vi "Main.vi"(11 "Module Admin":refnum<class "Delacor_lib_QMH_Module Admin.lvclass">) -> ()   [LabVIEW 2020, in "Cycling by State module.lvlib"]
doc: "This template is based off of the Queued Message Handler design pattern and the Queued Message Handler project template that ships with LabVIEW.\n\nThe main difference is that the queue is private to this module and communication between modules is performed via Broadcast and Request events.\n\nRequest events are wrapped in public API methods and are handled in the Event Handling Loop (EHL) of this VI. Any module can register for Broadcast events sent by this module. The EHL generates messages based on user interface actions.\n\nThe Message Handling Loop (MHL) processes messages generated by the EHL, or by other messages. The messages are string values, so new messages can be added easily to the Message Cases case structure in the MHL. Each message cluster can also provide an optional value for Message Data, which is a variant that can be converted to whatever message-specific data is required.\n_____\nBased on DQMH Project Template 7.0.1.1316."
uses:
  Cycling by State module.lvlib
  <vilib>/Delacor/Delacor QMH/Libraries/Module Admin_class/Delacor_lib_QMH_Module Admin.lvclass
  Module Data--cluster.ctl
  Cycling HL Data--cluster.ctl
  Cycling state.ctl
  <vilib>/Delacor/Delacor QMH/Libraries/Message Queue_class/Delacor_lib_QMH_Message Queue.lvclass/Delacor_lib_QMH_Message Queue.ctl
  Stop Argument--cluster.ctl
  <vilib>/Delacor/Delacor QMH/Libraries/Module Admin_class/Delacor_lib_QMH_Module Admin.lvclass/Delacor_lib_QMH_Module Admin.ctl
  Start cycling Argument--cluster.ctl
  Stop cycling Argument--cluster.ctl
  <vilib>/Utility/miscctls.llb/LVPointTypeDef.ctl
  <vilib>/Delacor/Delacor QMH/Libraries/Message Queue_class/Delacor_lib_QMH_Enqueue Message (Single).vi
  <vilib>/Delacor/Delacor QMH/Libraries/Module Admin_class/Delacor_lib_QMH_Get External Launch.vi
  <vilib>/Delacor/Delacor QMH/Libraries/Message Queue_class/Delacor_lib_QMH_Message Queue.lvclass
  Sensor checking module/Sensor checking module.lvlib
panel:
  out "error out":errorcluster
  out "Status":string
  in  "Simulate MHL Error":bool
  in  "Simulate EHL Error":bool
  # "Other processes communicate with this Module via its Public API (wrappers for its Request Events).\n\nThis Module communicates with other processes via its Broadcast Events.\nAny process that wants to receive these messages can register for this module's Broadcast events."
  # "This template is for the DQMH framework. See the block diagram for more information on how to use this template."
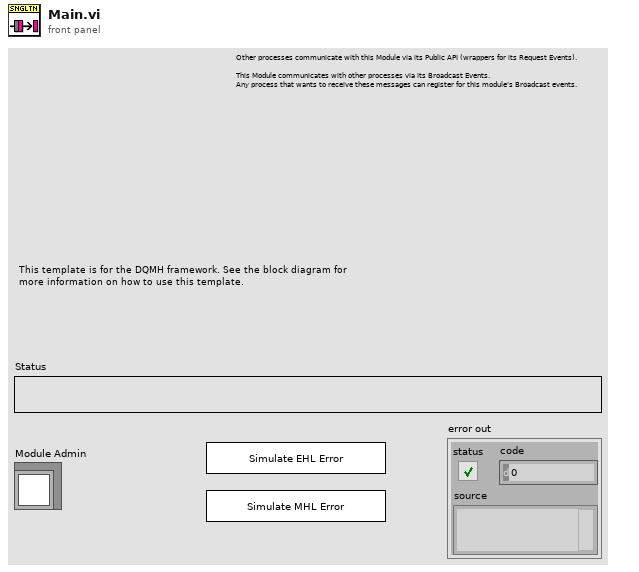
[diagram p1: front panel]
types:
  T1 = typedef "Cycling by State module.lvlib/Request Events--cluster.ctl" = cluster{"Stop Module":refnum<user-event>, "Show Panel":refnum<user-event>, "Hide Panel":refnum<user-event>, "Get Module Execution Status":refnum<user-event>, "Show Diagram":refnum<user-event>, "Start cycling":refnum<user-event>, "Stop cycling":refnum<user-event>, "Private":cluster{"Wake up cycling HL":refnum<user-event>}, "Put Cycling HL to sleep":refnum<user-event>}
  T2 = typedef "Sensor checking module.lvlib/Broadcast Events--cluster.ctl" = cluster{"Module Did Init":refnum<user-event>, "Status Updated":refnum<user-event>, "Error Reported":refnum<user-event>, "Module Did Stop":refnum<user-event>, "Update Module Execution Status":refnum<user-event>, "Triggered Broadcast":refnum<user-event>}
  T3 = typedef "Cycling by State module.lvlib/Cycling HL Data--cluster.ctl" = cluster{"Enum":T4, "RPM":dbl, "Triggered interval":dbl}
  T4 = typedef "Cycling state.ctl" = enum16{"Accelerating to 110rpm", "Detecting 100rpm", "Pressing until 0rpm"}
  T5 = typedef "Cycling by State module.lvlib/Module Data--cluster.ctl" = cluster{"Status":string}
  T6 = enum32{"invalid lock state", "Not Locked", "Locked (No Password)", "Password-protected"}
  T7 = typedef "Cycling by State module.lvlib/Stop Argument--cluster.ctl" = cluster{"Origin":string, "Exit via Stop Module Req?":bool, "Wait for Module to stop?":bool}
  T8 = typedef "Cycling by State module.lvlib/Start cycling Argument--cluster.ctl" = cluster{"Triggered interval":dbl, "Cycling interval":dbl}
  T9 = typedef "Cycling by State module.lvlib/Stop cycling Argument--cluster.ctl" = cluster{"Boolean":bool}
  T10 = typedef "LVPointTypeDef.ctl" = cluster{"Horizontal":i16, "Vertical":i16}
  T11 = enum32{"Invalid", "Standard", "Closed", "Hidden", "Minimized", "Maximized"}
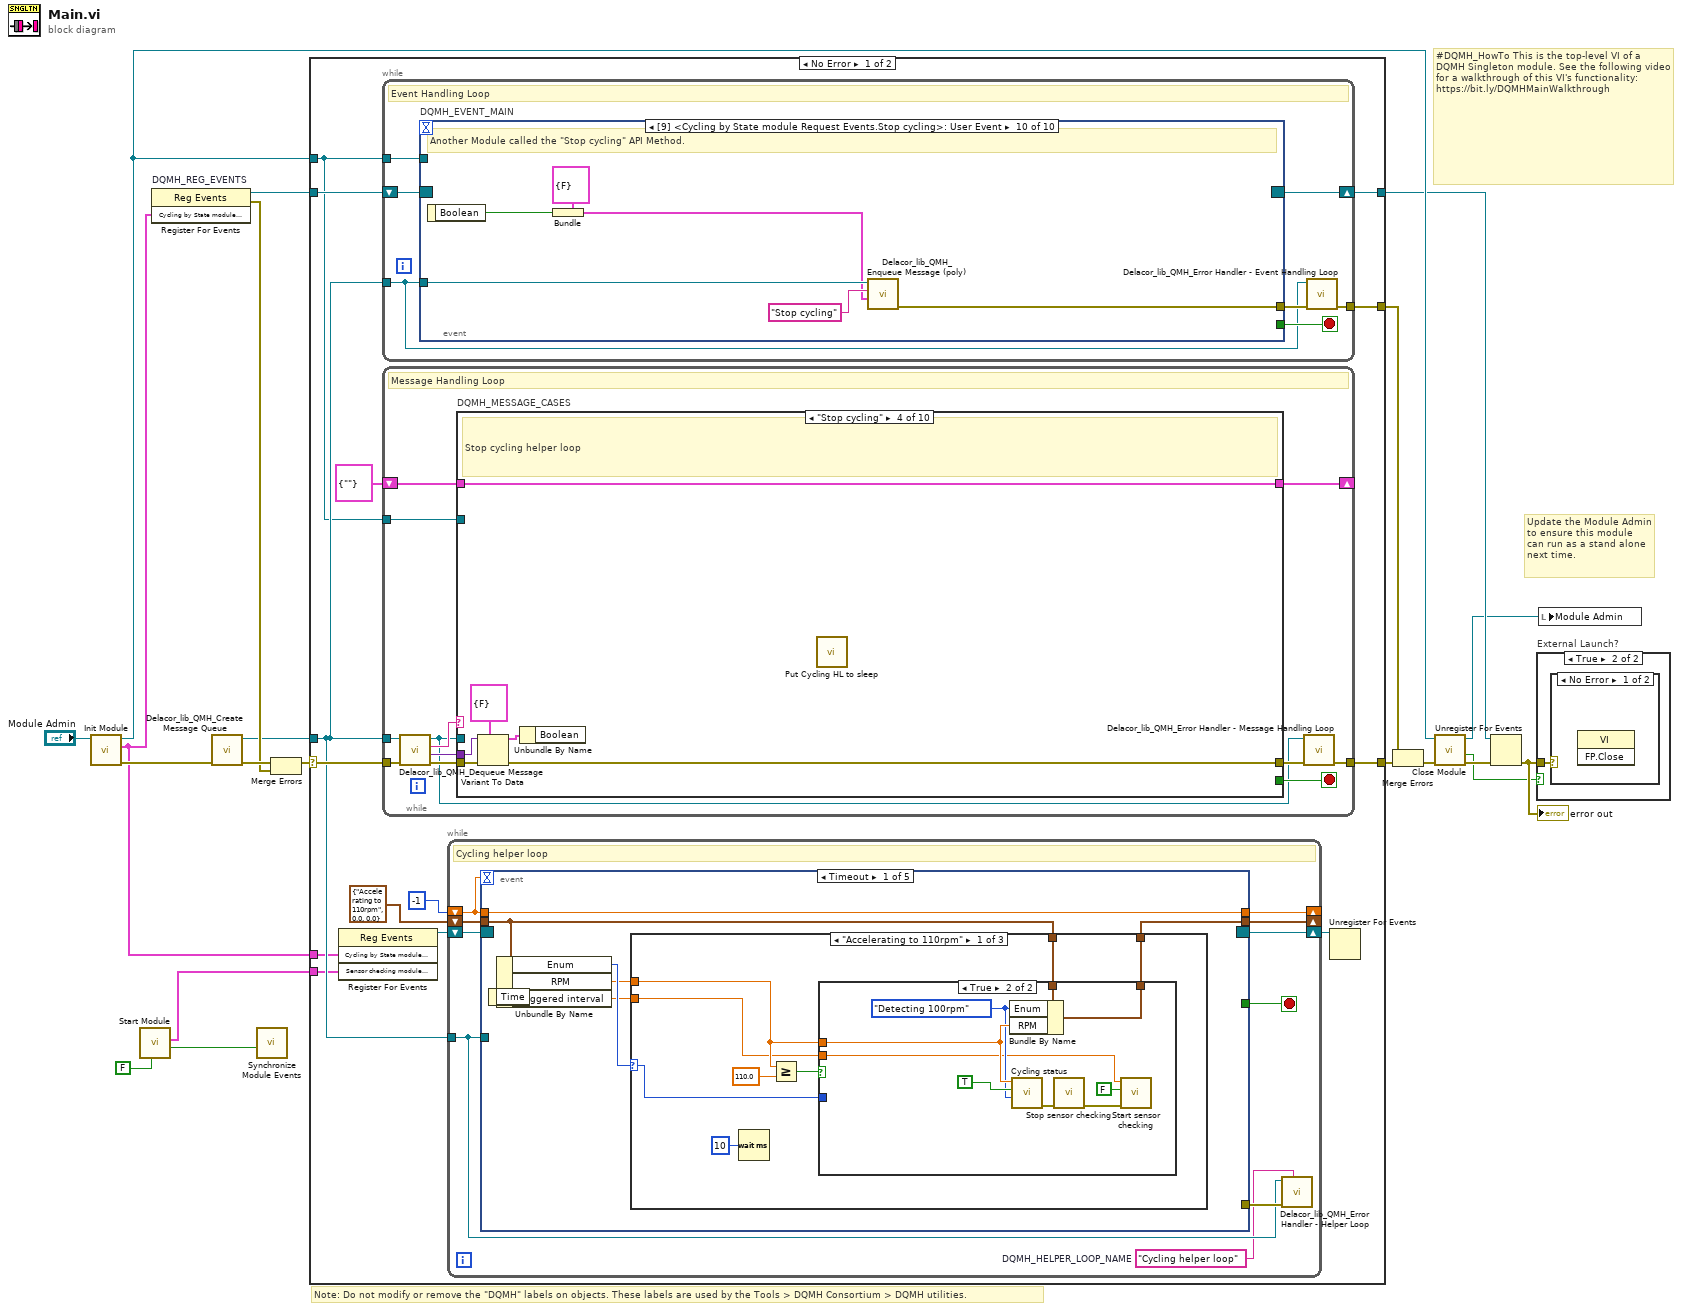
[diagram p0: block diagram]
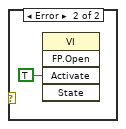
[diagram p3: hidden frame]
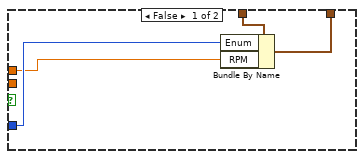
[diagram p4: hidden frame]
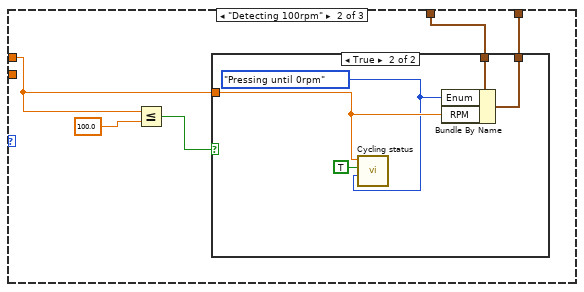
[diagram p5: hidden frame]
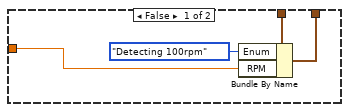
[diagram p6: hidden frame]
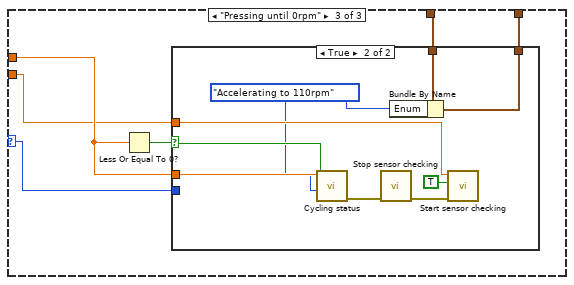
[diagram p7: hidden frame]
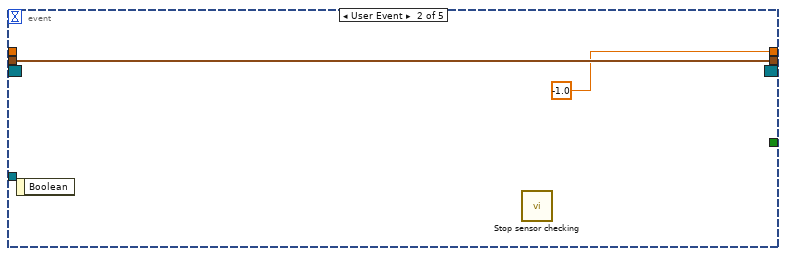
[diagram p9: hidden frame]
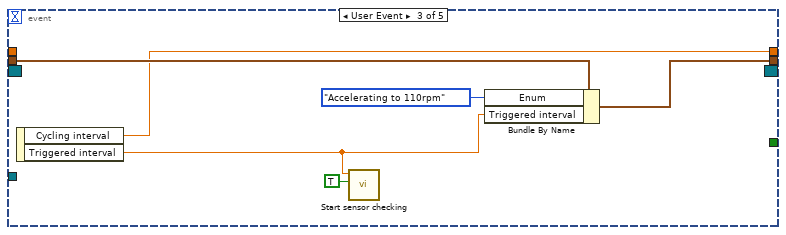
[diagram p10: hidden frame]
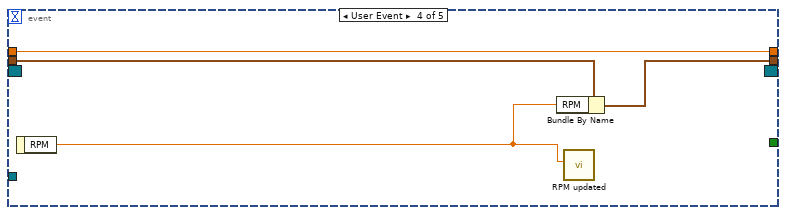
[diagram p11: hidden frame]
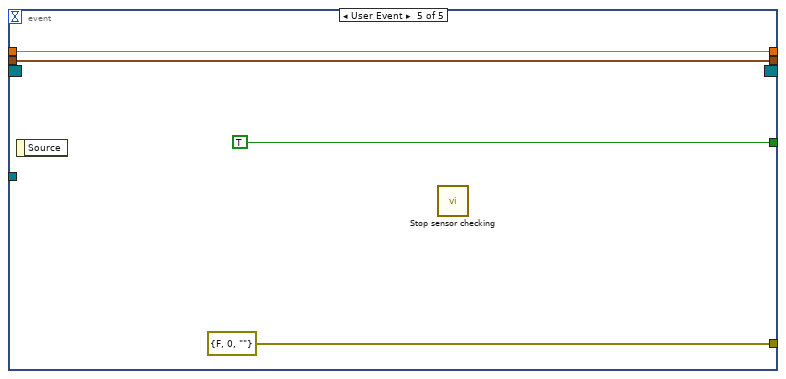
[diagram p12: hidden frame]
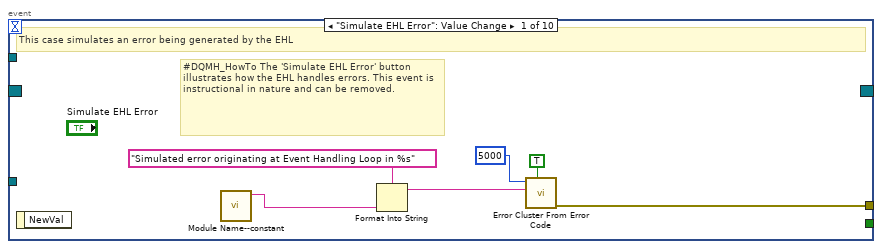
[diagram p13: hidden frame]
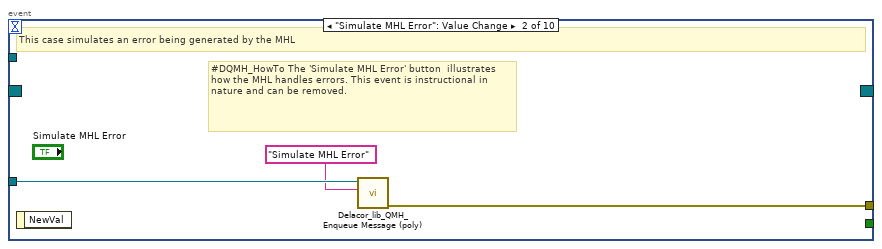
[diagram p14: hidden frame]
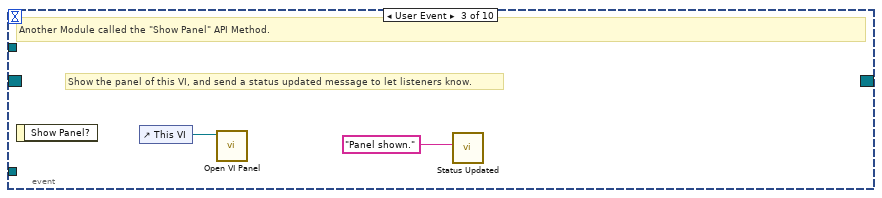
[diagram p15: hidden frame]
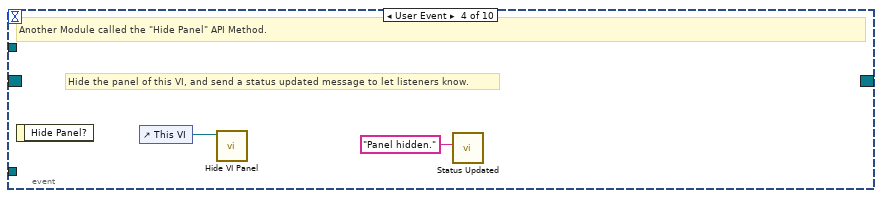
[diagram p16: hidden frame]
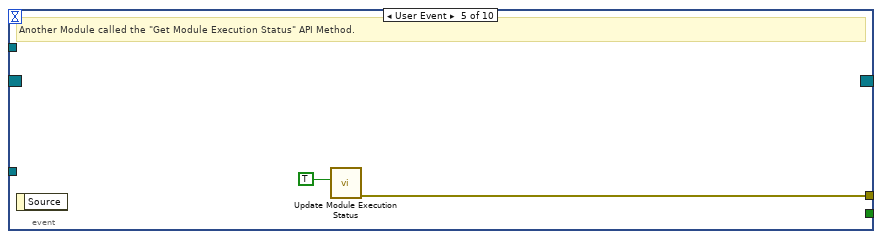
[diagram p17: hidden frame]
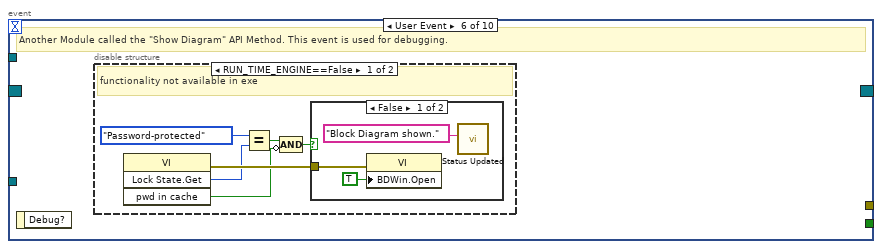
[diagram p18: hidden frame]
diagram:
  # "#DQMH_HowTo This is the top-level VI of a DQMH Singleton module. See the following video for a walkthrough of this VI's functionality: https://bit.ly/DQMHMainWalkthrough"
  # "Note: Do not modify or remove the \"DQMH\" labels on objects. These labels are used by the Tools > DQMH Consortium > DQMH utilities."
  # "Update the Module Admin to ensure this module can run as a stand alone next time."
  n1 = call "Init Module.vi"("Singleton Module Admin in"="Module Admin") -> ("error out"=w19:errorcluster, "Cycling by State module Request Events"=w3:T1, "Singleton Module Admin out"=w11:refnum<class "Delacor_lib_QMH_Module Admin.lvclass">)  [unwired: 8 in]
  n2 = call "Start Module.vi"("Show Main VI Diagram on Init (F)"=FALSE) -> ("Wait for Event Sync?"=w1:bool, "Sensor checking module Broadcast Events"=w2:T2)  [unwired: 7 in, 2 out]
  n3 = register-events "DQMH_REG_EVENTS"(w3) -> (reference out=w9:refnum<event-registration>, error out=w12:errorcluster)  [unwired: 2 in]
  n4 = call <vilib>:"Delacor_lib_QMH_Create Message Queue.vi"("error in"=w19) -> ("error out"=w14:errorcluster, "Message Queue"=w8:refnum<class "Delacor_lib_QMH_Message Queue.lvclass">)  [unwired: 9 in]
  n5 = call "Synchronize Module Events.vi"("Wait for Event Sync?"=w1) -> ()  [unwired: 10 in, 1 out]
  n6 = Merge Errors(w14, w12) -> (w13:errorcluster)
  n7 = case shown="No Error" w13 {
    selector: w13 -> [w32 w297]
    tunnel: [w34 w296] -> w20
    tunnel: [w31 w295] -> w10
    tunnel: w9 -> [w29 w295]
    tunnel: w8 -> [w28 w290]
    tunnel: [w33 _] -> w17
    tunnel: w11 -> [w27 w291]
    tunnel: w3 -> [w26 _]
    tunnel: w2 -> [w22 _]
    frame No Error {
      n8 = register-events ("DQMH_HELPER_REGFOREVENTS")(w26, w22) -> (reference out=w24:refnum<event-registration>)  [unwired: 2 in, 1 out]
      n9 = while {
        tunnel: w28 -> [w118]
        shift-right: [w121] -> w31
        shift-left: w29 -> [w122]
        tunnel: [w123] -> w33
        tunnel: w27 -> [w119]
        stop <- w120 stop-if-true
        # "Event Handling Loop"
        n10 = event "DQMH_EVENT_MAIN" shown="[9] <Cycling by State module Request Events.Stop cycling>: User Event" {
          selector: w122 -> [_ _ _ _ _ _ _ _ _ _]
          dyn-events: [_ _ _ _ _ _ _ _ _ _] -> w121
          timeout: _ -> [_ _ _ _ _ _ _ _ _ _]
          tunnel: [_ _ _ _ _ _ TRUE ("Discard?") _ _ _] -> w120
          tunnel: w118 -> [_ w132 _ _ _ _ w156 w163 w179 w185]
          tunnel: [w130 w133 _ _ w139 _ w159 w165 w174 w180] -> w124
          tunnel: w119 -> [_ _ _ _ _ _ _ w162 _ _]
          event "Simulate EHL Error": Value Change {
            # "#DQMH_HowTo The 'Simulate EHL Error' button  illustrates how the EHL handles errors. This event is instructional in nature and can be removed."
            # "This case simulates an error being generated by the EHL"
            n11 = event-data() -> ()  [unwired: 1 in, 1 out]
            n12 = call "Module Name--constant.vi"() -> ("Module Name"=w127:string)  [unwired: 11 in]
            n13 = Format Into String(format string="Simulated error originating at Event Handling Loop in %s", w127) -> (resulting string=w128:string)  [unwired: 2 in, 1 out]
            n14 = call <vilib>:"Error Cluster From Error Code.vi"("show call chain? (False)"=TRUE, "error message (\"\")"=w128, "error code (0)"=5000) -> ("error out"=w130:errorcluster)  [unwired: 6 in]
          }
          event "Simulate MHL Error": Value Change {
            # "#DQMH_HowTo The 'Simulate MHL Error' button  illustrates how the MHL handles errors. This event is instructional in nature and can be removed."
            # "This case simulates an error being generated by the MHL"
            n15 = event-data() -> ()  [unwired: 1 in, 1 out]
            n16 = call-poly <vilib>:"Delacor_lib_QMH_Enqueue Message (poly).vi"("Message"="Simulate MHL Error", "Message Queue in"=w132) -> ("error out"=w133:errorcluster)  [unwired: 8 in, 1 out]
          }
          event User Event {
            # "Show the panel of this VI, and send a status updated message to let listeners know."
            # "Another Module called the \"Show Panel\" API Method."
            n17 = event-data() -> ()  [unwired: 1 in, 1 out]
            n18 = control-ref of="This VI"() -> (w135:refnum<vi>)
            n19 = call "Open VI Panel.vi"("VI"=w135) -> ()  [unwired: 10 in, 1 out]
            n20 = call "Status Updated.vi"("Status"="Panel shown." ("format string")) -> ()  [unwired: 10 in, 1 out]
          }
          event User Event {
            # "Hide the panel of this VI, and send a status updated message to let listeners know."
            # "Another Module called the \"Hide Panel\" API Method."
            n21 = event-data() -> ()  [unwired: 1 in, 1 out]
            n22 = control-ref of="This VI"() -> (w137:refnum<vi>)
            n23 = call "Hide VI Panel.vi"("VI"=w137) -> ()  [unwired: 10 in, 1 out]
            n24 = call "Status Updated.vi"("Status"="Panel hidden." ("format string")) -> ()  [unwired: 10 in, 1 out]
          }
          event User Event {
            # "Another Module called the \"Get Module Execution Status\" API Method."
            n25 = event-data() -> ()  [unwired: 1 in, 1 out]
            n26 = call "Update Module Execution Status.vi"("Running?"=TRUE) -> ("error out"=w139:errorcluster)  [unwired: 10 in]
          }
          event User Event {
            # "Another Module called the \"Show Diagram\" API Method. This event is used for debugging."
            n27 = event-data() -> ()  [unwired: 1 in, 1 out]
            n28 = disable-structure shown="RUN_TIME_ENGINE==False" {
              frame condition #0 (active) {
                # "functionality not available in exe"
                n29 = invoke on="Invoke Node" class="VI" method="Lock State.Get"() -> (error out=w145:errorcluster, "Get Lock State"=w144:T6, "pwd in cache"=w141:bool)  [unwired: 4 in, 1 out]
                n30 = Equal?(x=T6."Password-protected", y=w144) -> (x = y?=w142:bool)
                n31 = Compound Arithmetic op=AND(w142, invert w141) -> (w140:bool)
                n32 = case shown="False" w140 {
                  tunnel: w145 -> [w148 _]
                  frame False {
                    n33 = property on="Property Node" class="VI"(error in=w148, "BDWin.Open"=TRUE ("Block Diagram Window:Open")) -> ()  [unwired: 1 in, 2 out]
                    n34 = call "Status Updated.vi"("Status"="Block Diagram shown." ("format string")) -> ()  [unwired: 10 in, 1 out]
                  }
                  frame True {
                    # "Password-protected VI, and the password is not in the cache. Do not show the diagram."
                  }
                }
              }
              frame condition #1 {
              }
            }
          }
          event User Event {
            # "The Stop Module Event can get fired from the Exit message in the MHL. The queue gets destroyed in that case. If the queue no longer exists, the Enqueue Exit as a priority message will return error 1. It is safe to ignore, because the module is already exiting."
            # "Another Module called the \"Stop Module\" API Method  or the Message Handling Loop below."
            n35 = event-data() -> ("Origin"=w155:string, "Exit via Stop Module Req?"=w151:bool, "Wait for Module to stop?"=w150:bool)  [unwired: 1 in]
            n36 = local write "Status"(w155) -> ()
            n37 = Bundle By Name(cluster=T7 {"Origin"="", "Exit via Stop Module Req?"=FALSE, "Wait for Module to stop?"=FALSE} ("Stop Argument"), "Exit via Stop Module Req?"=w151, "Wait for Module to stop?"=w150) -> (w149:T7)
            n38 = call-poly <vilib>:"Delacor_lib_QMH_Enqueue Message (poly).vi"("Priority Message? (F)"=TRUE, "Message Data"=w149, "Message"="Exit", "Message Queue in"=w156) -> ("error out"=w160:errorcluster)  [unwired: 6 in, 1 out]
            n39 = call <vilib>:"Clear Errors.vi"("error in (no error)"=w160, "specific error code to clear (0: all)"=1) -> ("error out"=w159:errorcluster)  [unwired: 4 in, 1 out]
          }
          event Panel Close? {
            w164 = TRUE  # Discard the event, the MHL is responsible for closing and stopping this VI.
            # "Hide the panel or send the 'Exit' message if the user clicks the 'X' on the module main VI panel."
            n40 = event-data() -> ()  [unwired: 1 in, 1 out]
            n41 = property on="Property Node" class="Module Admin"(reference=w162) -> ("Accessors:External Launch"=w161:bool)  [unwired: 1 in, 2 out]
            n42 = case shown="True" w161 {
              tunnel: w163 -> [_ w171]
              tunnel: [_ w172] -> w165
              frame True {
                # "If externally launched, clicking the 'X' hides the panel, but doesn't close it."
                n43 = control-ref of="This VI"() -> (w168:refnum<vi>)
                n44 = call "Hide VI Panel.vi"("VI"=w168) -> ("error out"=w166:errorcluster)  [unwired: 10 in]
                n45 = call "Status Updated.vi"("error in"=w166, "Status"="Panel hidden." ("format string")) -> ()  [unwired: 9 in, 1 out]
              }
              frame False {
                # "If run as a stand-alone VI, clicking the panel 'X' stops the VI."
                n46 = call-poly <vilib>:"Delacor_lib_QMH_Enqueue Message (poly).vi"("Priority Message? (F)"=TRUE, "Message"="Exit", "Message Queue in"=w171) -> ("error out"=w172:errorcluster)  [unwired: 7 in, 1 out]
              }
            }
            n47 = event-data ("Event Filter Node")("Discard?"=w164) -> ()  [unwired: 1 in, 1 out]
          }
          event User Event {
            # "Another Module called the \"Start cycling\" API Method."
            n48 = event-data() -> ("Triggered interval"=w175:dbl, "Cycling interval"=w173:dbl)  [unwired: 1 in]
            n49 = Bundle(cluster=T8 {"Triggered interval"=500.0, "Cycling interval"=500.0} ("Start cycling Argument"), "Triggered interval"=w175, "Cycling interval"=w173) -> (w176:T8)
            n50 = call-poly <vilib>:"Delacor_lib_QMH_Enqueue Message (poly).vi"("Message Data"=w176, "Message"="Start cycling", "Message Queue in"=w179) -> ("error out"=w174:errorcluster)  [unwired: 7 in, 1 out]
          }
          event User Event {
            # "Another Module called the \"Stop cycling\" API Method."
            n51 = event-data() -> ("Boolean"=w181:bool)  [unwired: 1 in]
            n52 = Bundle(cluster=T9 {"Boolean"=FALSE} ("Stop cycling Argument"), "Boolean"=w181) -> (w182:T9)
            n53 = call-poly <vilib>:"Delacor_lib_QMH_Enqueue Message (poly).vi"("Message Data"=w182, "Message"="Stop cycling", "Message Queue in"=w185) -> ("error out"=w180:errorcluster)  [unwired: 7 in, 1 out]
          }
        }
        n54 = call-dynamic "Delacor_lib_QMH_Error Handler - Event Handling Loop.vi"("error in"=w124, "Message Queue in"=w118) -> ("dup error in"=w123:errorcluster)  [unwired: 8 in, 1 out]
      }
      n55 = while {
        tunnel: w28 -> [w186]
        shift-right: [w194] -> _
        shift-left: T5 {"Status"=""} ("Data Cluster") -> [w195]
        tunnel: w32 -> [w197]
        tunnel: [w189] -> w34
        tunnel: w27 -> [w190]
        stop <- w193 stop-if-true
        # "Message Handling Loop"
        n56 = call-dynamic "Delacor_lib_QMH_Dequeue Message.vi"("error in"=w197, "Message Queue in"=w186) -> ("error out"=w196:errorcluster, "Message Data"=w191:variant, "Message"=w192:string, "Message Queue out"=w187:refnum<class "Delacor_lib_QMH_Message Queue.lvclass">)  [unwired: 6 in]
        n57 = case "DQMH_MESSAGE_CASES" shown="\"Stop cycling\"" w192 {
          selector: w192 -> [_ _ _ _ _ _ _ _ _ w285]
          tunnel: w187 -> [_ _ _ _ _ _ _ w251 w273 _]
          tunnel: w196 -> [w215 w219 w227 w233 w236 w238 w247 w258 w279 w288]
          tunnel: [w213 w219 w225 w231 w235 w238 w246 w254 w274 w289] -> w188
          tunnel: w195 -> [w204 w218 w226 w232 w234 w237 w244 w253 w272 w286]
          tunnel: [w203 w218 w226 w232 w234 w237 w244 w253 w272 w286] -> w194
          tunnel: [_ _ _ _ _ _ _ _ w271 _] -> w193
          tunnel: w191 -> [_ _ w224 w230 _ _ _ w252 w270 _]
          tunnel: w190 -> [w205 _ _ _ _ _ _ w250 w265 _]
          frame "Initialize" {
            w199 = "Initial Message" ("Initial Message")
            # "#CodeNeeded - Initialize the appearance of the front panel."
            # "#CodeNeeded - Initialize your state data here."
            # "Initialize - Any operation that needs to be done before the module can receive messages. Synchronize Caller Events.vi will inform Start Module.vi that the module has launched and is ready to receive messages. Module Did Init.vi will broadcast that the module initialized."
            n58 = call "Synchronize Caller Events.vi"("error in"=w215, "Singleton Module Admin in"=w205) -> ("error out"=w214:errorcluster, "Singleton Module Admin out"=w200:refnum<class "Delacor_lib_QMH_Module Admin.lvclass">)  [unwired: 8 in]
            n59 = property on="Property Node" class="Module Admin"(reference=w200) -> ("Accessors:External Launch"=w209:bool)  [unwired: 1 in, 2 out]
            n60 = Select(t=T11."Hidden" ("State"), s=w209, f=T11."Standard" ("State")) -> (s? t:f=w206:T11)
            n61 = call "Module Name--constant.vi"() -> ("Module Name"=w212:string)  [unwired: 11 in]
            n62 = property on="Property Node" class="VI"("Front Panel.Title"=w212) -> (reference out=w211:refnum<vi>, error out=w217:errorcluster)  [unwired: 2 in]
            n63 = call "Module Name--constant.vi"() -> ("Module Name"=w201:string)  [unwired: 11 in]
            n64 = invoke on="Invoke Node" class="VI" method="FP.Open"(reference=w211, error in=w217, "State"=w206) -> (reference out=w210:refnum<vi>, error out=w216:errorcluster)  [unwired: 2 in, 3 out]
            n65 = Bundle By Name(cluster=w204, "Status"=w199) -> (w203:T5)
            n66 = call "Module Did Init.vi"("error in"=w214, "Initialized?"=TRUE, "Origin"=w201) -> ("error out"=w213:errorcluster)  [unwired: 8 in]
            n67 = invoke on="Invoke Node" class="VI" method="FP.Center"(reference=w210, error in=w216) -> ()  [unwired: 1 in, 3 out]
            n68 = property on="Pane" class="Pane"("Origin"=T10 {"Horizontal"=0, "Vertical"=0}) -> ()  [unwired: 2 in, 2 out]
            "Status" <- w199
          }
          frame "---Module Specific---" {
            # "Separator -- The following cases handle messages specific to this Module."
          }
          frame "Start cycling" {
            # "To start cycling by waking up cycling helper loop"
            n69 = Variant To Data(error in=w227, type=T8 {"Triggered interval"=500.0, "Cycling interval"=500.0} ("Start cycling Argument"), Variant=w224) -> (data=w222:T8, error out=w225:errorcluster)
            n70 = Unbundle By Name(w222) -> ("Triggered interval"=w221:dbl, "Cycling interval"=w220:dbl)
            n71 = call "Wake up cycling HL.vi"("Triggered interval"=w221, "Cycling interval"=w220) -> ()  [unwired: 8 in, 1 out]
          }
          frame "Stop cycling" {
            # "Stop cycling helper loop"
            n72 = Variant To Data(error in=w233, type=T9 {"Boolean"=FALSE} ("Stop cycling Argument"), Variant=w230) -> (data=w228:T9, error out=w231:errorcluster)
            n73 = Unbundle By Name(w228) -> ()  [unwired: 1 out]
            n74 = call "Put Cycling HL to sleep.vi"() -> ()  [unwired: 11 in, 1 out]
          }
          frame "---Copy This Frame---" {
            # "Duplicate this frame when creating new messages.  Change this comment in the duplicated frame to describe this message."
            n75 = Merge Errors(w236) -> (w235:errorcluster)
          }
          frame "---Exit and Error Handling---" {
            # "Separator - The following cases handle errors and exit messages."
          }
          frame "Simulate MHL Error" {
            # "#DQMH_HowTo The 'Simulate MHL Error' button  illustrates how the MHL handles errors. This event is instructional in nature and can be removed."
            # "Simulate an error occurring at the MHL"
            n76 = call "Module Name--constant.vi"() -> ("Module Name"=w240:string)  [unwired: 11 in]
            n77 = Format Into String(format string="Simulated error originating at Message Handling Loop in %s", w240) -> (resulting string=w241:string)  [unwired: 2 in, 1 out]
            n78 = call <vilib>:"Error Cluster From Error Code.vi"("show call chain? (False)"=TRUE, "error message (\"\")"=w241, "error code (0)"=5001) -> ("error out"=w245:errorcluster)  [unwired: 6 in]
            n79 = Merge Errors(w247, w245) -> (w246:errorcluster)
          }
          frame "Error" {
            # "#CodeRecommended - If the module is running in standalone mode (External Launch = FALSE), this code will pop up an error dialog and call the 'Exit' message if an error occurs. Add more fine-grained error management here."
            # "Error - Check the error message data and respond accordingly. This message is sent by the \"Error Handler\" VIs at the end of each loop in this application."
            n80 = property on="Property Node" class="Module Admin"(reference=w250) -> ("Accessors:External Launch"=w249:bool)  [unwired: 1 in, 2 out]
            n81 = Variant To Data(error in=w258, type=errorcluster {"status"=FALSE, "code"=0, "source"=""} ("error constant"), Variant=w252) -> (data=w248:errorcluster, error out=w256:errorcluster)
            n82 = local write "error out"(w248) -> ()
            n83 = call "Error Reported.vi"("Error"=w248) -> ()  [unwired: 10 in, 1 out]
            n84 = case shown="False" w249 {
              tunnel: [w263 _] -> w255
              tunnel: w251 -> [w261 _]
              tunnel: w248 -> [w262 _]
              frame False {
                n85 = disable-structure shown="Default" {
                  disable-tunnel: w262 -> [w264 _]
                  frame condition #0 (active) {
                    # "If the module is running standalone, then pop up an error dialog and call the \"Exit\" message."
                    n86 = call <vilib>:"Simple Error Handler.vi"("error in (no error)"=w264) -> ()  [unwired: 4 in, 5 out]
                  }
                  frame condition #1 {
                    # "To prevent the Simple Error Handler VI from being loaded (e.g. when deploying to a Real-Time target), add the Conditional Disable Symbol \"DQMH_Disable_SEH\" to your project and set it to TRUE."
                  }
                }
                n87 = call-poly <vilib>:"Delacor_lib_QMH_Enqueue Message (poly).vi"("Priority Message? (F)"=TRUE, "Message"="Exit", "Message Queue in"=w261) -> ("error out"=w263:errorcluster)  [unwired: 7 in, 1 out]
              }
              frame True {
                # "If the module was launched externally, calling the Error Reported broadcast VI is the only action performed by the \"Error\" message. The module's caller can then process the error appropriately."
              }
            }
            n88 = Merge Errors(w256, w255) -> (w254:errorcluster)
          }
          frame "Exit" {
            w269 = 91  # 91: not all Exit messages will have an argument
            w271 = TRUE  # Stop the VI
            # "Release the message queue reference"
            # "#CodeNeeded - Add any required cleanup code here."
            # "Exit - Exit the application."
            n89 = Variant To Data(error in=w279, type=T7 {"Origin"="", "Exit via Stop Module Req?"=FALSE, "Wait for Module to stop?"=FALSE} ("Stop Argument"), Variant=w270) -> (data=w267:T7, error out=w276:errorcluster)
            n90 = call <vilib>:"Clear Errors.vi"("error in (no error)"=w276, "specific error code to clear (0: all)"=w269) -> ("error out"=w278:errorcluster)  [unwired: 4 in, 1 out]
            n91 = control-ref of="This VI"() -> (w266:refnum<vi>)
            n92 = call-dynamic "Delacor_lib_QMH_Release Message Queue.vi"("error in"=w278, "Message Queue"=w273) -> ("error out"=w277:errorcluster)  [unwired: 9 in]
            n93 = call "Handle Exit.vi"("Stop Argument"=w267, "Admin in"=w265, "VI reference"=w266) -> ("error out"=w275:errorcluster)  [unwired: 7 in, 1 out]
            n94 = Merge Errors(w277, w275) -> (w274:errorcluster)
            n95 = call "Error Reported.vi"("Error"=w274) -> ()  [unwired: 10 in, 1 out]
            n96 = call "Stop Module.vi"() -> ()  [unwired: 11 in, 1 out]
          }
          frame Default {
            # "'Default' case only runs if there is a message that isn't defined in any of the other cases.  Output a programming error."
            n97 = call "Module Name--constant.vi"() -> ("Module Name"=w284:string)  [unwired: 11 in]
            n98 = Format Into String(format string="The invalid message string \"%s\" was received in the Message Handling Loop for module \"%s\".", w285, w284) -> (resulting string=w280:string)  [unwired: 2 in, 1 out]
            n99 = call <vilib>:"Error Cluster From Error Code.vi"("show call chain? (False)"=TRUE, "error message (\"\")"=w280, "error code (0)"=1) -> ("error out"=w287:errorcluster)  [unwired: 6 in]
            n100 = Merge Errors(w288, w287) -> (w289:errorcluster)
          }
        }
        n101 = call-dynamic "Delacor_lib_QMH_Error Handler - Message Handling Loop.vi"("error in"=w188, "Message Queue in"=w187) -> ("dup error in"=w189:errorcluster)  [unwired: 8 in, 1 out]
      }
      n102 = while "DQMH_HELPER_LOOP" {
        shift-right: [w44] -> _
        shift-left: -1 -> [w43]
        shift-right: [w41] -> w25
        shift-left: w24 -> [w42]
        tunnel: w28 -> [w38]
        shift-right: [w35] -> _
        shift-left: T3 {"Enum"=enum."Accelerating to 110rpm", "RPM"=0.0, "Triggered interval"=0.0} ("Cycling HL Data") -> [w36]
        stop <- w40 stop-if-true
        w37 = "Cycling helper loop"  # DQMH_HELPER_LOOP_NAME
        # "Cycling helper loop"
        n103 = event "DQMH_HELPER_EVENT_STRUCTURE" shown="[0] Timeout" {
          selector: w42 -> [_ _ _ _ _]
          dyn-events: [_ _ _ _ _] -> w41
          timeout: w43 -> [_ _ _ _ _]
          tunnel: w43 -> [w50 _ _ w113 w117]
          tunnel: [w50 -1.0 ("Cycling interval") w106 w113 w117] -> w44
          tunnel: [_ _ _ _ TRUE] -> w40
          tunnel: [_ _ _ _ errorcluster {"status"=FALSE, "code"=0, "source"=""} ("error constant")] -> w39
          tunnel: w38 -> [_ _ _ _ _]
          tunnel: w36 -> [w48 w103 w109 w111 w114]
          tunnel: [w47 w103 w108 w112 w114] -> w35
          event Timeout {
            n104 = event-data() -> ()  [unwired: 1 in, 1 out]
            n105 = Unbundle By Name(w48) -> ("Enum"=w49:T4, "RPM"=w46:dbl, "Triggered interval"=w45:dbl)
            n106 = case shown="\"Accelerating to 110rpm\"" w49 {
              selector: w49 -> [w55 _ w91]
              tunnel: w48 -> [w58 w72 w89]
              tunnel: [w57 w73 w90] -> w47
              tunnel: w46 -> [w54 w74 w87]
              tunnel: w45 -> [w52 _ w86]
              frame "Accelerating to 110rpm" {
                n107 = Wait (ms)(milliseconds to wait=u32 10) -> ()  [unwired: 1 out]
                n108 = Greater Or Equal?(x=w54, y=110.0) -> (x >= y?=w53:bool)
                n109 = case shown="True" w53 {
                  tunnel: w58 -> [w59 w71]
                  tunnel: [w60 w70] -> w57
                  tunnel: w55 -> [w62 _]
                  tunnel: w54 -> [w61 w68]
                  tunnel: w52 -> [_ w63]
                  frame False {
                    n110 = Bundle By Name(cluster=w59, "Enum"=w62, "RPM"=w61) -> (w60:T3)
                  }
                  frame True {
                    w67 = Cycling_state."Detecting 100rpm" ("Enum")
                    n111 = Bundle By Name(cluster=w71, "Enum"=w67, "RPM"=w68) -> (w70:T3)
                    n112 = call "Cycling status.vi"("Enum"=w67, "Triggered?"=TRUE, "RPM"=w68) -> ("error out"=w66:errorcluster)  [unwired: 8 in]
                    n113 = call "Stop sensor checking.vi"("error in"=w66) -> ("error out"=w65:errorcluster)  [unwired: 10 in]
                    n114 = call "Start sensor checking.vi"("Triggered interval"=w63, "RPM increasing?"=FALSE, "error in"=w65) -> ()  [unwired: 7 in, 1 out]
                  }
                }
              }
              frame "Detecting 100rpm" {
                n115 = Less Or Equal?(x=w74, y=100.0) -> (x <= y?=w75:bool)
                n116 = case shown="True" w75 {
                  tunnel: w74 -> [w77 w82]
                  tunnel: [w79 w84] -> w73
                  tunnel: w72 -> [w80 w83]
                  frame False {
                    n117 = Bundle By Name(cluster=w80, "Enum"=Cycling_state."Detecting 100rpm", "RPM"=w77) -> (w79:T3)
                  }
                  frame True {
                    w81 = Cycling_state."Pressing until 0rpm" ("Enum")
                    n118 = call "Cycling status.vi"("Enum"=w81, "Triggered?"=TRUE, "RPM"=w82) -> ()  [unwired: 8 in, 1 out]
                    n119 = Bundle By Name(cluster=w83, "Enum"=w81, "RPM"=w82) -> (w84:T3)
                  }
                }
              }
              frame "Pressing until 0rpm" {
                n120 = Less Or Equal To 0?(x=w87) -> (x <= 0?=w88:bool)
                n121 = case shown="True" w88 {
                  selector: w88 -> [_ w101]
                  tunnel: w91 -> [_ _]
                  tunnel: [w92 w100] -> w90
                  tunnel: w89 -> [w92 w99]
                  tunnel: w87 -> [_ w98]
                  tunnel: w86 -> [_ w94]
                  frame False {
                  }
                  frame True {
                    w93 = Cycling_state."Accelerating to 110rpm" ("Enum")
                    n122 = call "Cycling status.vi"("Enum"=w93, "Triggered?"=w101, "RPM"=w98) -> ("error out"=w95:errorcluster)  [unwired: 8 in]
                    n123 = call "Stop sensor checking.vi"("error in"=w95) -> ("error out"=w97:errorcluster)  [unwired: 10 in]
                    n124 = Bundle By Name(cluster=w99, "Enum"=w93) -> (w100:T3)
                    n125 = call "Start sensor checking.vi"("Triggered interval"=w94, "RPM increasing?"=TRUE, "error in"=w97) -> ()  [unwired: 7 in, 1 out]
                  }
                }
              }
            }
          }
          event User Event {
            n126 = event-data() -> ()  [unwired: 1 in, 1 out]
            n127 = call "Stop sensor checking.vi"() -> ()  [unwired: 11 in, 1 out]
          }
          event User Event {
            n128 = event-data() -> ("Cycling interval"=w106:dbl, "Triggered interval"=w104:dbl)  [unwired: 1 in]
            n129 = call "Start sensor checking.vi"("Triggered interval"=w104, "RPM increasing?"=TRUE) -> ()  [unwired: 8 in, 1 out]
            n130 = Bundle By Name(cluster=w109, "Enum"=Cycling_state."Accelerating to 110rpm", "Triggered interval"=w104) -> (w108:T3)
          }
          event User Event {
            n131 = event-data() -> ("RPM"=w110:dbl)  [unwired: 1 in]
            n132 = Bundle By Name(cluster=w111, "RPM"=w110) -> (w112:T3)
            n133 = call "RPM updated.vi"("RPM"=w110) -> ()  [unwired: 10 in, 1 out]
          }
          event User Event {
            n134 = event-data() -> ()  [unwired: 1 in, 1 out]
            n135 = call "Stop sensor checking.vi"() -> ()  [unwired: 11 in, 1 out]
          }
        }
        n136 = call-dynamic "Delacor_lib_QMH_Error Handler - Helper Loop.vi"("Error Debug"=w37, "error in"=w39, "Message Queue in"=w38) -> ()  [unwired: 7 in, 2 out]
      }
      n137 = Unregister For Events(event registration refnum=w25) -> ()  [unwired: 1 in, 1 out]
    }
    frame Error {
      # "Synchronize Caller Events.vi will inform Start Module.vi that the module has launched and will let the code calling Start Module.vi register for broadcasts and would permit the caller receive the broadcast that an error occurred at launch time."
      n138 = call-dynamic "Delacor_lib_QMH_Release Message Queue.vi"("error in"=w297, "Message Queue"=w290) -> ("error out"=w296:errorcluster)  [unwired: 9 in]
      n139 = call "Synchronize Caller Events.vi"("Singleton Module Admin in"=w291) -> ("error out"=w298:errorcluster)  [unwired: 9 in, 1 out]
      n140 = call "Module Name--constant.vi"() -> ("Module Name"=w294:string)  [unwired: 11 in]
      n141 = Format Into String(format string="An error occurred during initialization. %s is no longer running.", w294) -> (resulting string=w292:string)  [unwired: 2 in, 1 out]
      n142 = Merge Errors(w296, w298) -> (w299:errorcluster)
      n143 = call "Error Reported.vi"("Additional Information"=w292, "Error"=w299) -> ()  [unwired: 9 in, 1 out]
    }
  }
  n144 = Merge Errors(w17, w20) -> (w16:errorcluster)
  n145 = call "Close Module.vi"("error in"=w16, "Module Admin in"=w11) -> ("error out"=w18:errorcluster, "External Launch"=w5:bool, "Module Admin out"=w6:refnum<class "Delacor_lib_QMH_Module Admin.lvclass">)  [unwired: 7 in]
  n146 = Unregister For Events(event registration refnum=w10, error in=w18) -> (error out=w15:errorcluster)
  "error out" <- w15
  n147 = case "External Launch?" shown="True" w5 {
    tunnel: w15 -> [_ w300]
    frame False {
    }
    frame True {
      n148 = case shown="No Error" w300 {
        frame No Error {
          n149 = invoke on="Invoke Node" class="VI" method="FP.Close"() -> ()  [unwired: 3 in, 3 out]
        }
        frame Error {
          n150 = invoke on="Invoke Node" class="VI" method="FP.Open"("Activate"=TRUE ("Activate?")) -> ()  [unwired: 4 in, 5 out]
        }
      }
    }
  }
  n151 = local write "Module Admin"(w6) -> ()
